vi "Periodic Tasks.vi"(8 "error in":errorcluster) -> ()   [LabVIEW 2015]
doc: "This VI runs in parallel to other tasks. It can contain as many user-defined periodic loops as you need. These can carry out PID or other sorts of timed response."
uses:
  <vilib>/Rock Robotics/WPI/Solenoid/WPI_SolenoidValue.ctl
  <vilib>/Rock Robotics/WPI/Utilities/WPI_GetSetVariantRefNum.vi
  Robot Global Data.vi
  <vilib>/addons/control/pid/pid.llb/PID (DBL).vi
  <vilib>/Rock Robotics/WPI/Solenoid/WPI_SolenoidSetEnum.vi
  <vilib>/addons/control/pid/NI_PID_pid.lvlib
panel:
  out "LeftInches":dbl
  out "RightInches":dbl
  out "Encoder1 Rate":dbl
  out "Encoder2 Rate":dbl
  in  "PID gains Up":T1={"proportional gain (Kc)"=1.0, "integral time (Ti, min)"=0.01, "derivative time (Td, min)"=0.0}
  in  "PID gains down":T1={"proportional gain (Kc)"=1.0, "integral time (Ti, min)"=0.01, "derivative time (Td, min)"=0.0}
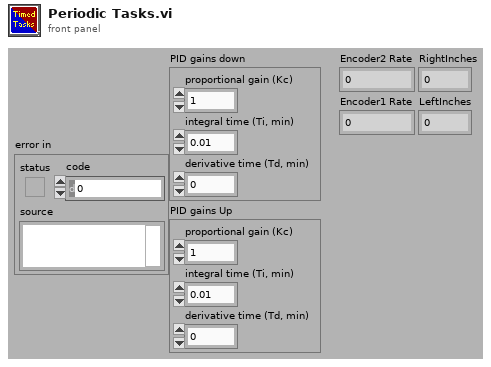
[diagram p1: front panel]
types:
  T1 = cluster{"proportional gain (Kc)":dbl, "integral time (Ti, min)":dbl, "derivative time (Td, min)":dbl}
  T2 = typedef "WPI_EncoderDevRef.ctl" = cluster{"DevStatus":errorcluster, "EncoderIndex":T3, "CounterIndex":T4, "DistancePerCount":dbl, "Decoding Type":T5}
  T3 = typedef "FPGA_EncoderIdx.ctl" = enum8{"Enc 0", "Enc 1", "Enc 2", "Enc 3", "Enc 4", "Enc 5", "Enc 6", "Enc 7", "Invalid"}
  T4 = typedef "FPGA_CounterCtrSystemIndex.ctl" = enum8{"Ctr 0", "Ctr 1", "Ctr 2", "Ctr 3", "Ctr 4", "Ctr 5", "Ctr 6", "Ctr 7", "Invalid"}
  T5 = typedef "WPI_EncoderType.ctl" = enum16{"1x", "2x", "4x"}
  T6 = typedef "WPI_ServoDeviceRef.ctl" = cluster{"DeviceStatus":errorcluster, "PWM Channel":T7, "DeadBand":T8}
  T7 = typedef "FPGA_DIOPWMChannel.ctl" = enum8{"PWM 0", "PWM 1", "PWM 2", "PWM 3", "PWM 4", "PWM 5", "PWM 6", "PWM 7", "PWM 8", "PWM 9", "PWM MXP 0", "PWM MXP 1", "PWM MXP 2", "PWM MXP 3", "PWM MXP 4", "PWM MXP 5", "PWM MXP 6", "PWM MXP 7", "PWM MXP 8", "PWM MXP 9", "Invalid"}
  T8 = typedef "WPI_PWMDeadband.ctl" = cluster{"Name":string, "maxPositivePwm":i32, "minPositivePwm":i32, "centerPwm":i32, "maxNegativePwm":i32, "minNegativePwm":i32, "angularRange":u16}
  T9 = typedef "WPI_SolenoidDevRef.ctl" = cluster{"DevStatus":errorcluster, "Pneumatics Control Module":u8, "Forward Solenoid Channel":T10, "Reverse Solenoid Channel":T10}
  T10 = typedef "WPI_SolenoidChannel.ctl" = enum8{"Solenoid 0", "Solenoid 1", "Solenoid 2", "Solenoid 3", "Solenoid 4", "Solenoid 5", "Solenoid 6", "Solenoid 7", "Invalid"}
  T11 = typedef "WPI_PotentiometerDevRef.ctl" = cluster{"DevStatus":errorcluster, "Analog Channel":T12, "Invert Output":bool}
  T12 = typedef "FPGA_AIChannel.ctl" = enum8{"AI 0", "AI 1", "AI 2", "AI 3", "AI MXP 0", "AI MXP 1", "AI MXP 2", "AI MXP 3", "Invalid"}
  T13 = typedef "WPI_MotorControlDeviceRef.ctl" = cluster{"DeviceStatus":errorcluster, "Type":T14, "PWM":cluster{"PWM Channel":T7, "DeadBand":T8}, "CAN":cluster{"Device Number":u8, "Control Mode":T15, "Semaphore":T16, "Max Vout":dbl, "TalonSRX Control Mode":T17}, "Invert":bool}
  T14 = typedef "WPI_MotorControlType.ctl" = enum16{"PWM", "CAN", "CANTalonSRX"}
  T15 = typedef "WPI_CANJaguar_ControlMode.ctl" = enum8{"Percent VBus", "Current", "Speed", "Position", "Voltage"}
  T16 = typedef "Semaphore RefNum" = refnum<k1>
  T17 = typedef "WPI_CANTalonSRX_APIControlMode.ctl" = enum8{"Percent VBus", "Speed", "Position", "Slave", "Unchanged / Invalid", "Voltage Compensation", "Current", "Motion Profile"}
  T18 = typedef "WPI_JoystickDevRef.ctl" = cluster{"Device":T19}
  T19 = typedef "WPI_JoystickDeviceEnum.ctl" = enum16{"USB 0", "USB 1", "USB 2", "USB 3", "USB 4", "USB 5"}
  T20 = typedef "WPI_SolenoidValue.ctl" = enum16{"Off", "On", "Forward", "Reverse"}
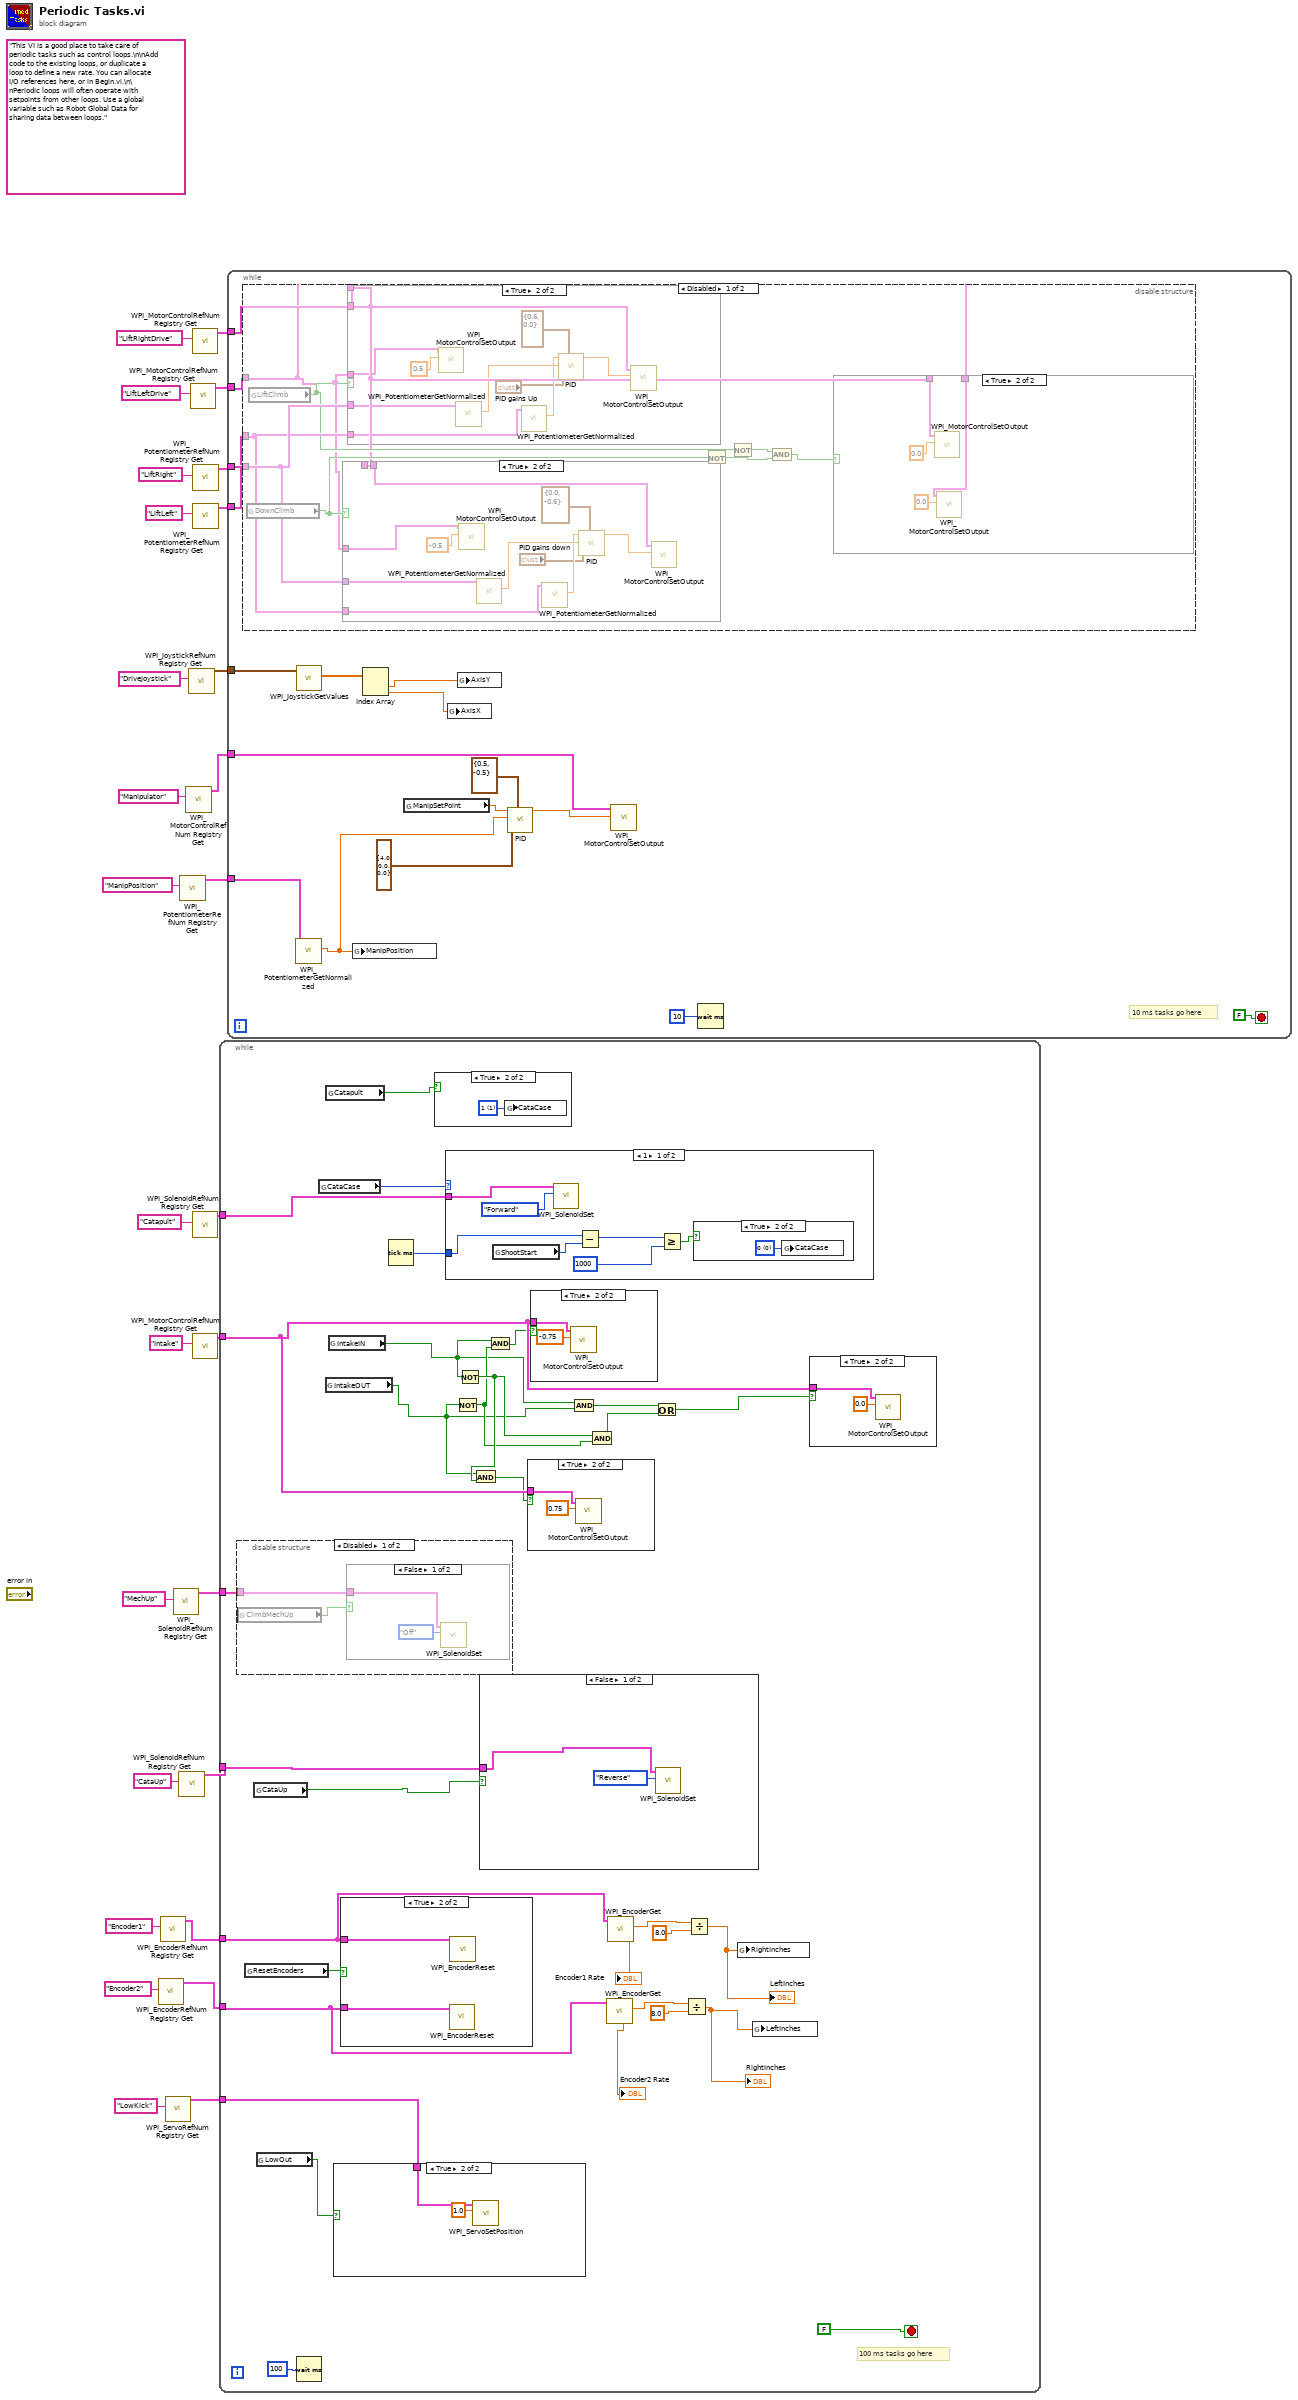
[diagram p0: block diagram]
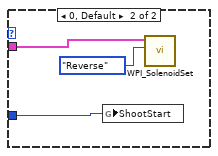
[diagram p4: hidden frame]
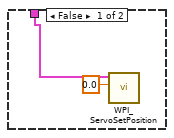
[diagram p5: hidden frame]
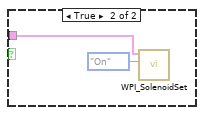
[diagram p6: hidden frame]
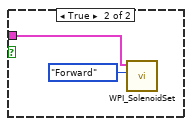
[diagram p12: hidden frame]
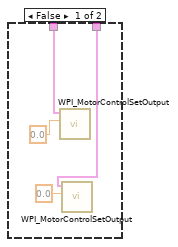
[diagram p14: hidden frame]
diagram:
  (unwired) "This VI is a good place to take care of periodic tasks such as control loops.\n\nAdd code to the existing loops, or duplicate a loop to define a new rate. You can allocate I/O references here, or in Begin.vi.\n\nPeriodic loops will often operate with setpoints from other loops. Use a global variable such as Robot Global Data for sharing data between loops."
  n1 = call <vilib>:"WPI_EncoderRefNum Registry Get.vi"("refnum name"="Encoder2") -> ("EncoderDevRef"=w8:T2)  [unwired: 9 in, 1 out]
  n2 = call <vilib>:"WPI_EncoderRefNum Registry Get.vi"("refnum name"="Encoder1") -> ("EncoderDevRef"=w7:T2)  [unwired: 9 in, 1 out]
  n3 = call <vilib>:"WPI_ServoRefNum Registry Get.vi"("refnum name"="LowKick") -> ("ServoDeviceRef"=w1:T6)  [unwired: 9 in, 1 out]
  n4 = call <vilib>:"WPI_SolenoidRefNum Registry Get.vi"("refnum name"="MechUp") -> ("SolenoidDevRef"=w16:T9)  [unwired: 9 in, 1 out]
  n5 = call <vilib>:"WPI_SolenoidRefNum Registry Get.vi"("refnum name"="CataUp") -> ("SolenoidDevRef"=w13:T9)  [unwired: 9 in, 1 out]
  n6 = call <vilib>:"WPI_PotentiometerRefNum Registry Get.vi"("refnum name"="ManipPosition") -> ("PotDevRef"=w5:T11)  [unwired: 9 in, 1 out]
  n7 = call <vilib>:"WPI_MotorControlRefNum Registry Get.vi"("refnum name"="Manipulator") -> ("MotorControlDevRef"=w3:T13)  [unwired: 9 in, 1 out]
  n8 = call <vilib>:"WPI_JoystickRefNum Registry Get.vi"("refnum name"="DriveJoystick") -> ("JoystickDevRef"=w11:T18)  [unwired: 9 in, 1 out]
  n9 = call <vilib>:"WPI_MotorControlRefNum Registry Get.vi"("refnum name"="LiftLeftDrive") -> ("MotorControlDevRef"=w15:T13)  [unwired: 9 in, 1 out]
  n10 = call <vilib>:"WPI_MotorControlRefNum Registry Get.vi"("refnum name"="LiftRightDrive") -> ("MotorControlDevRef"=w20:T13)  [unwired: 9 in, 1 out]
  n11 = call <vilib>:"WPI_SolenoidRefNum Registry Get.vi"("refnum name"="Catapult") -> ("SolenoidDevRef"=w27:T9)  [unwired: 9 in, 1 out]
  n12 = call <vilib>:"WPI_MotorControlRefNum Registry Get.vi"("refnum name"="Intake") -> ("MotorControlDevRef"=w25:T13)  [unwired: 9 in, 1 out]
  n13 = call <vilib>:"WPI_PotentiometerRefNum Registry Get.vi"("refnum name"="LiftRight") -> ("PotDevRef"=w18:T11)  [unwired: 9 in, 1 out]
  n14 = call <vilib>:"WPI_PotentiometerRefNum Registry Get.vi"("refnum name"="LiftLeft") -> ("PotDevRef"=w19:T11)  [unwired: 9 in, 1 out]
  n15 = while {
    tunnel: w27 -> [w58]
    tunnel: w25 -> [w45]
    tunnel: w16 -> [w57]
    tunnel: w13 -> [w35]
    tunnel: w8 -> [w54]
    tunnel: w7 -> [w55]
    tunnel: w1 -> [w32]
    stop <- FALSE stop-if-true
    # "100 ms tasks go here"
    n16 = disable-structure shown="Disabled" {
      disable-tunnel: w57 -> [w78 _]
      frame Disabled {
        n17 = global read "Robot Global Data.vi" "ClimbMechUp"() -> (w77:bool)
        n18 = case shown="False" w77 {
          tunnel: w78 -> [w79 w82]
          frame False {
            n19 = call-poly <vilib>:"WPI_SolenoidSet.vi"("Value"=WPI_SolenoidValue."Off", "SolenoidDevRef"=w79) -> ()  [unwired: 8 in, 2 out]
          }
          frame True {
            n20 = call-poly <vilib>:"WPI_SolenoidSet.vi"("Value"=WPI_SolenoidValue."On", "SolenoidDevRef"=w82) -> ()  [unwired: 8 in, 2 out]
          }
        }
      }
      frame Enabled {
      }
    }
    n21 = global read "Robot Global Data.vi" "ResetEncoders"() -> (w56:bool)
    n22 = global read "Robot Global Data.vi" "CataUp"() -> (w34:bool)
    n23 = global read "Robot Global Data.vi" "LowOut"() -> (w33:bool)
    n24 = Wait (ms)(milliseconds to wait=u32 100) -> ()  [unwired: 1 out]
    n25 = global read "Robot Global Data.vi" "CataCase"() -> (w31:u16)
    n26 = global read "Robot Global Data.vi" "IntakeOUT"() -> (w37:bool)
    n27 = global read "Robot Global Data.vi" "Catapult"() -> (w30:bool)
    n28 = global read "Robot Global Data.vi" "IntakeIN"() -> (w38:bool)
    n29 = case shown="True" w33 {
      tunnel: w32 -> [w73 w75]
      frame False {
        n30 = call <vilib>:"WPI_ServoSetPosition.vi"("Position"=0.0, "ServoDeviceRef"=w73) -> ()  [unwired: 8 in, 2 out]
      }
      frame True {
        n31 = call <vilib>:"WPI_ServoSetPosition.vi"("Position"=1.0, "ServoDeviceRef"=w75) -> ()  [unwired: 8 in, 2 out]
      }
    }
    n32 = case shown="True" w56 {
      tunnel: w54 -> [_ w90]
      tunnel: w55 -> [_ w89]
      frame False {
      }
      frame True {
        n33 = call <vilib>:"WPI_EncoderReset.vi"("EncoderDevRef"=w90) -> ()  [unwired: 9 in, 2 out]
        n34 = call <vilib>:"WPI_EncoderReset.vi"("EncoderDevRef"=w89) -> ()  [unwired: 9 in, 2 out]
      }
    }
    n35 = Tick Count (ms)() -> (millisecond timer value=w29:u32)
    n36 = case shown="True" w30 {
      frame False {
      }
      frame True {
        w61 = u16 1 items=["0", "1"] ("CataCase")
        n37 = global write "Robot Global Data.vi" "CataCase"(w61) -> ()
      }
    }
    n38 = case shown="1" w31 {
      tunnel: w58 -> [w67 w72]
      tunnel: w29 -> [w66 w70]
      frame 1 {
        n39 = global read "Robot Global Data.vi" "ShootStart"() -> (w65:u32)
        n40 = call-poly <vilib>:"WPI_SolenoidSet.vi"("Value"=WPI_SolenoidValue."Forward", "SolenoidDevRef"=w67) -> ()  [unwired: 8 in, 2 out]
        n41 = Subtract(x=w66, y=w65) -> (x-y=w64:u32)
        n42 = Greater Or Equal?(x=w64, y=u32 1000 ("ShootDelay")) -> (x >= y?=w63:bool)
        n43 = case shown="True" w63 {
          frame False {
          }
          frame True {
            w69 = u16 0 items=["0", "1"] ("CataCase")
            n44 = global write "Robot Global Data.vi" "CataCase"(w69) -> ()
          }
        }
      }
      frame 0, Default {
        n45 = global write "Robot Global Data.vi" "ShootStart"(w70) -> ()
        n46 = call-poly <vilib>:"WPI_SolenoidSet.vi"("Value"=WPI_SolenoidValue."Reverse", "SolenoidDevRef"=w72) -> ()  [unwired: 8 in, 2 out]
      }
    }
    n47 = Not(x=w37) -> (.not. x?=w41:bool)
    n48 = Not(x=w38) -> (.not. x?=w43:bool)
    n49 = And(x=w37, y=w43) -> (x .and. y?=w44:bool)
    n50 = case shown="False" w34 {
      tunnel: w35 -> [w91 w93]
      frame False {
        n51 = call-poly <vilib>:"WPI_SolenoidSet.vi"("Value"=WPI_SolenoidValue."Reverse", "SolenoidDevRef"=w91) -> ()  [unwired: 8 in, 2 out]
      }
      frame True {
        n52 = call-poly <vilib>:"WPI_SolenoidSet.vi"("Value"=WPI_SolenoidValue."Forward", "SolenoidDevRef"=w93) -> ()  [unwired: 8 in, 2 out]
      }
    }
    n53 = And(x=w38, y=w41) -> (x .and. y?=w42:bool)
    n54 = case shown="True" w44 {
      tunnel: w45 -> [_ w86]
      frame False {
      }
      frame True {
        n55 = call <vilib>:"WPI_MotorControlSetOutput.vi"("Output"=0.75, "MotorControlDevRef"=w86) -> ()  [unwired: 7 in, 3 out]
      }
    }
    n56 = case shown="True" w42 {
      tunnel: w45 -> [_ w88]
      frame False {
      }
      frame True {
        n57 = call <vilib>:"WPI_MotorControlSetOutput.vi"("Output"=-0.75, "MotorControlDevRef"=w88) -> ()  [unwired: 7 in, 3 out]
      }
    }
    n58 = And(x=w38, y=w37) -> (x .and. y?=w39:bool)
    n59 = And(x=w43, y=w41) -> (x .and. y?=w40:bool)
    n60 = call <vilib>:"WPI_EncoderGet.vi"("EncoderDevRef"=w54) -> ("Distance"=w50:dbl, "Rate"=→"Encoder2 Rate":dbl)  [unwired: 5 in, 4 out]
    n61 = call <vilib>:"WPI_EncoderGet.vi"("EncoderDevRef"=w55) -> ("Distance"=w48:dbl, "Rate"=→"Encoder1 Rate":dbl)  [unwired: 5 in, 4 out]
    n62 = Or(x=w39, y=w40) -> (x .or. y?=w36:bool)
    n63 = Divide(x=w50, y=8.0) -> (x/y=w46:dbl)
    "RightInches" <- w46
    n64 = Divide(x=w48, y=8.0) -> (x/y=w47:dbl)
    "LeftInches" <- w47
    n65 = global write "Robot Global Data.vi" "RightInches"(w47) -> ()
    n66 = global write "Robot Global Data.vi" "LeftInches"(w46) -> ()
    n67 = case shown="True" w36 {
      tunnel: w45 -> [_ w84]
      frame False {
      }
      frame True {
        n68 = call <vilib>:"WPI_MotorControlSetOutput.vi"("Output"=0.0, "MotorControlDevRef"=w84) -> ()  [unwired: 7 in, 3 out]
      }
    }
  }
  n69 = while {
    tunnel: w20 -> [w103]
    tunnel: w19 -> [w108]
    tunnel: w18 -> [w109]
    tunnel: w15 -> [w102]
    tunnel: w11 -> [w106]
    tunnel: w5 -> [w101]
    tunnel: w3 -> [w100]
    stop <- FALSE stop-if-true
    # "10 ms tasks go here"
    n70 = disable-structure shown="Disabled" {
      disable-tunnel: w109 -> [w120 _]
      disable-tunnel: w108 -> [w119 _]
      disable-tunnel: w103 -> [w113 _]
      disable-tunnel: w102 -> [w112 _]
      frame Disabled {
        n71 = global read "Robot Global Data.vi" "DownClimb"() -> (w116:bool)
        n72 = global read "Robot Global Data.vi" "LiftClimb"() -> (w117:bool)
        n73 = case shown="True" w116 {
          tunnel: w113 -> [_ w124]
          tunnel: w112 -> [_ w123]
          tunnel: w120 -> [_ w122]
          tunnel: w119 -> [_ w121]
          tunnel: w113 -> [_ _]
          frame False {
          }
          frame True {
            n74 = call <vilib>:"WPI_MotorControlSetOutput.vi"("Output"=-0.5, "MotorControlDevRef"=w123) -> ()  [unwired: 7 in, 3 out]
            n75 = call <vilib>:"WPI_PotentiometerGetNormalized.vi"("PotDevRef"=w122) -> ("Normalized Value"=w129:dbl)  [unwired: 8 in, 2 out]
            n76 = call <vilib>:"WPI_PotentiometerGetNormalized.vi"("PotDevRef"=w121) -> ("Normalized Value"=w128:dbl)  [unwired: 8 in, 2 out]
            n77 = call-poly <vilib>:"PID.vi"("output range"=cluster{"output high":dbl, "output low":dbl} {"output high"=0.0, "output low"=-0.6}, "PID gains"="PID gains down", "process variable"=w129, "setpoint"=w128) -> ("output"=w125:dbl)  [unwired: 6 in, 1 out]
            n78 = call <vilib>:"WPI_MotorControlSetOutput.vi"("Output"=w125, "MotorControlDevRef"=w124) -> ()  [unwired: 7 in, 3 out]
          }
        }
        n79 = case shown="True" w117 {
          tunnel: w112 -> [_ w148]
          tunnel: w120 -> [_ w146]
          tunnel: w119 -> [_ w144]
          tunnel: w113 -> [_ w140]
          frame False {
          }
          frame True {
            n80 = call <vilib>:"WPI_MotorControlSetOutput.vi"("Output"=0.5, "MotorControlDevRef"=w148) -> ()  [unwired: 7 in, 3 out]
            n81 = call <vilib>:"WPI_PotentiometerGetNormalized.vi"("PotDevRef"=w146) -> ("Normalized Value"=w145:dbl)  [unwired: 8 in, 2 out]
            n82 = call <vilib>:"WPI_PotentiometerGetNormalized.vi"("PotDevRef"=w144) -> ("Normalized Value"=w143:dbl)  [unwired: 8 in, 2 out]
            n83 = call-poly <vilib>:"PID.vi"("output range"=cluster{"output high":dbl, "output low":dbl} {"output high"=0.6, "output low"=0.0}, "PID gains"="PID gains Up", "process variable"=w145, "setpoint"=w143) -> ("output"=w139:dbl)  [unwired: 6 in, 1 out]
            n84 = call <vilib>:"WPI_MotorControlSetOutput.vi"("Output"=w139, "MotorControlDevRef"=w140) -> ()  [unwired: 7 in, 3 out]
          }
        }
        n85 = Not(x=w116) -> (.not. x?=w114:bool)
        n86 = Not(x=w117) -> (.not. x?=w115:bool)
        n87 = And(x=w115, y=w114) -> (x .and. y?=w118:bool)
        n88 = case shown="True" w118 {
          tunnel: w113 -> [w131 w136]
          tunnel: w112 -> [w132 w135]
          frame False {
            n89 = call <vilib>:"WPI_MotorControlSetOutput.vi"("Output"=0.0, "MotorControlDevRef"=w131) -> ()  [unwired: 7 in, 3 out]
            n90 = call <vilib>:"WPI_MotorControlSetOutput.vi"("Output"=0.0, "MotorControlDevRef"=w132) -> ()  [unwired: 7 in, 3 out]
          }
          frame True {
            n91 = call <vilib>:"WPI_MotorControlSetOutput.vi"("Output"=0.0, "MotorControlDevRef"=w136) -> ()  [unwired: 7 in, 3 out]
            n92 = call <vilib>:"WPI_MotorControlSetOutput.vi"("Output"=0.0, "MotorControlDevRef"=w135) -> ()  [unwired: 7 in, 3 out]
          }
        }
      }
      frame Enabled {
      }
    }
    n93 = call <vilib>:"WPI_PotentiometerGetNormalized.vi"("PotDevRef"=w101) -> ("Normalized Value"=w98:dbl)  [unwired: 8 in, 2 out]
    n94 = call <vilib>:"WPI_JoystickGetValues.vi"("JoystickDevRef"=w106) -> ("Axes"=w107:dbl[])  [unwired: 6 in, 4 out]
    n95 = global write "Robot Global Data.vi" "ManipPosition"(w98) -> ()
    n96 = Index Array(array=w107) -> (element #1=w105:dbl, element #2=w104:dbl)  [unwired: 2 in]
    n97 = global read "Robot Global Data.vi" "ManipSetPoint"() -> (w99:dbl)
    n98 = global write "Robot Global Data.vi" "AxisX"(w104) -> ()
    n99 = global write "Robot Global Data.vi" "AxisY"(w105) -> ()
    n100 = call-poly <vilib>:"PID.vi"("output range"=cluster{"output high":dbl, "output low":dbl} {"output high"=0.5, "output low"=-0.5}, "PID gains"=T1 {"proportional gain (Kc)"=4.0, "integral time (Ti, min)"=0.0, "derivative time (Td, min)"=0.0}, "process variable"=w98, "setpoint"=w99) -> ("output"=w95:dbl)  [unwired: 6 in, 1 out]
    n101 = call <vilib>:"WPI_MotorControlSetOutput.vi"("Output"=w95, "MotorControlDevRef"=w100) -> ()  [unwired: 7 in, 3 out]
    n102 = Wait (ms)(milliseconds to wait=u32 10) -> ()  [unwired: 1 out]
  }
